vi "util_DoorInterface_cls_Is Door Open.vi"(0 "Interface_object in":refnum<class>, 5 "error in (no error)":errorcluster) -> (14 "Interface_object out":refnum<class>, 16 "Is Door Open?":bool, 19 "error out":errorcluster)   [LabVIEW 2018, in "Door.lvclass"]
uses:
  Door.lvclass
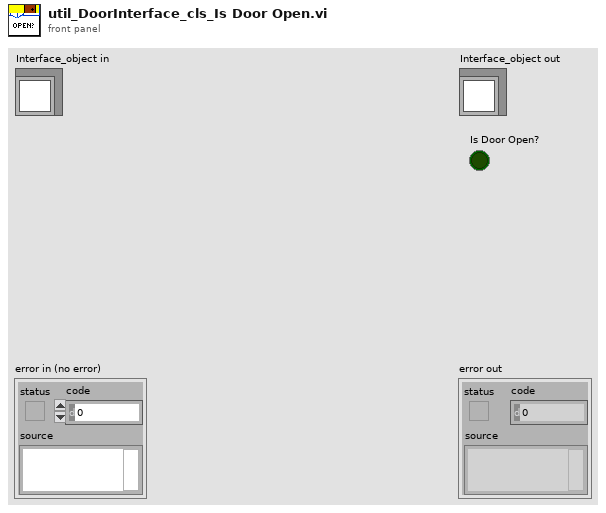
[diagram p1: front panel]
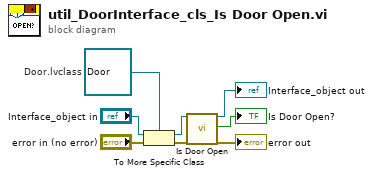
[diagram p0: block diagram]
diagram:
  w3 = refnum<class "Door.lvclass"> refnum  # Door.lvclass
  n1 = To More Specific Class(target class=w3, reference="Interface_object in", error in="error in (no error)") -> (specific class reference=w1:refnum<class "Door.lvclass">, error out=w2:errorcluster)
  n2 = call-dynamic "Is Door Open.vi"("Interface_object in"=w1, "error in (no error)"=w2) -> ("Interface_object out"=→"Interface_object out":refnum<class "Door.lvclass">, "Is Door Open?"=→"Is Door Open?":bool, "error out"=→"error out":errorcluster)  [unwired: 15 in]
